vi "CreateLocationNode.vi"(7 "DOM Document":refnum<k20>, 8 "Error In":errorcluster, 11 "Pattern":string) -> (0 "Error Out":errorcluster, 3 "Location Node":refnum<k20>)   [LabVIEW 2012]
uses:
  libs/LV-Utilities/LV-Utilities.lvlib
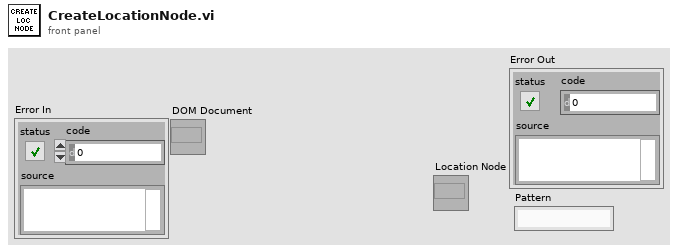
[diagram p1: front panel]
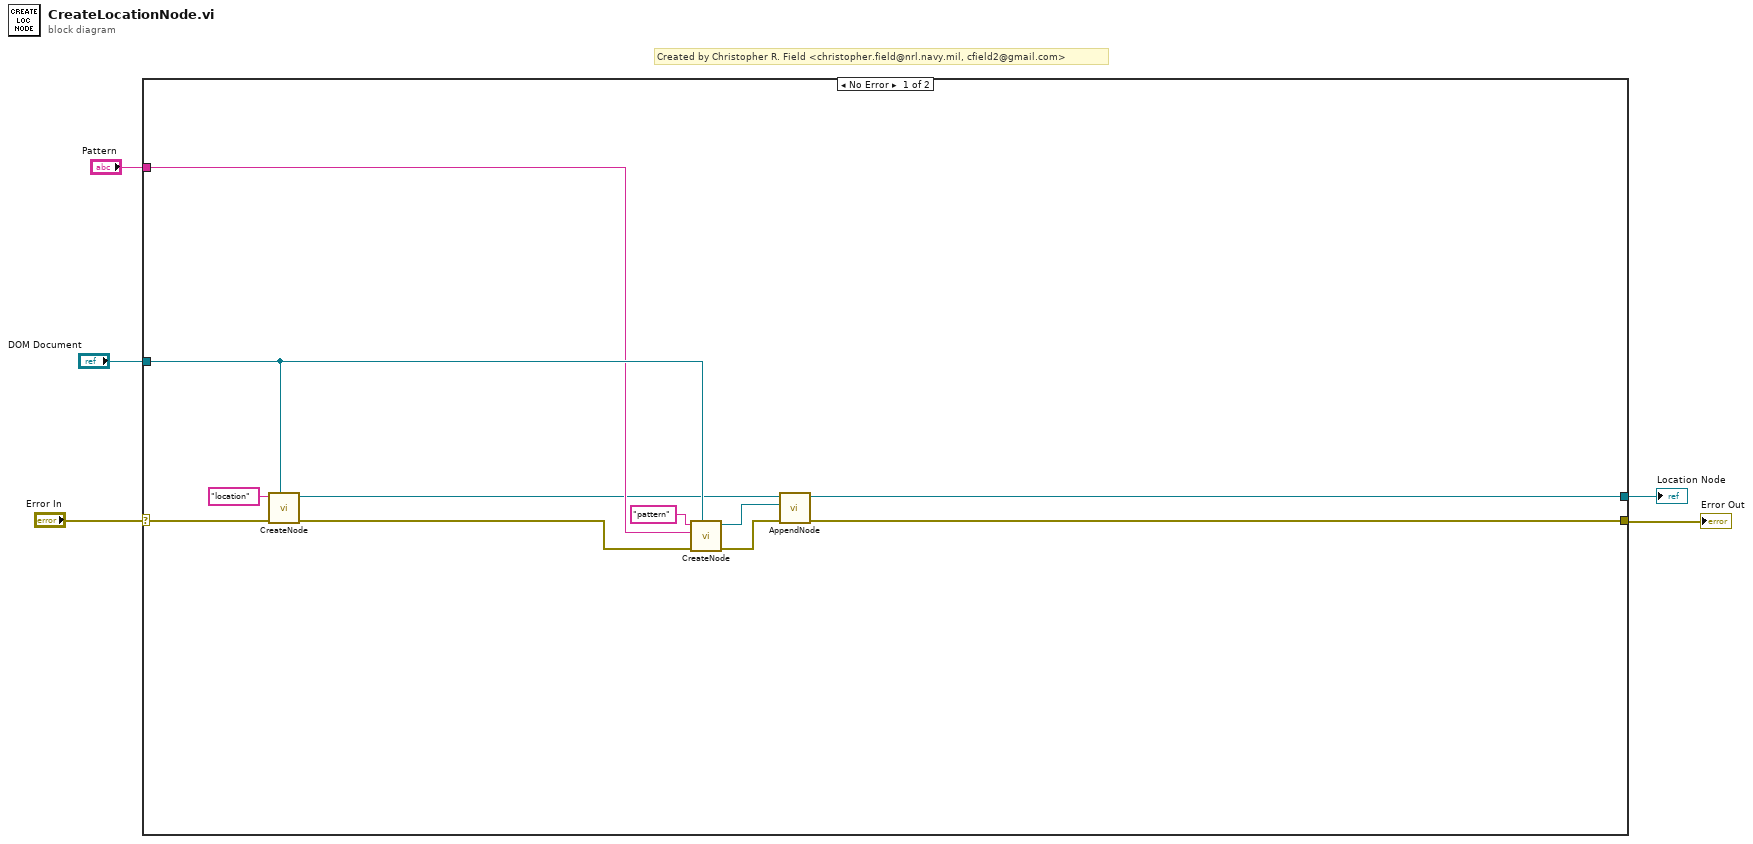
[diagram p0: block diagram]
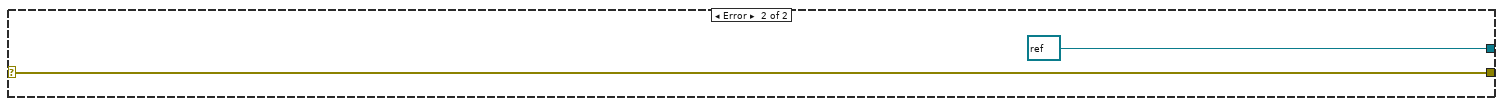
[diagram p2: hidden frame]
diagram:
  # "Created by Christopher R. Field <christopher.field@nrl.navy.mil, cfield2@gmail.com>"
  n1 = case shown="No Error" "Error In" {
    selector: "Error In" -> [w16 w18]
    tunnel: "DOM Document" -> [w14 _]
    tunnel: [w9 w18] -> w3
    tunnel: "Pattern" -> [w10 _]
    tunnel: [w8 refnum<k20> refnum ("Wirings Node 2")] -> w1
    frame No Error {
      n2 = call "CreateNode.vi"("DOM Document"=w14, "Error In"=w16, "Tag Name"="location") -> ("Error out"=w6:errorcluster, "Node"=w7:refnum<k20>)  [unwired: 7 in]
      n3 = call "CreateNode.vi"("DOM Document"=w14, "Error In"=w6, "Text"=w10, "Tag Name"="pattern") -> ("Error out"=w13:errorcluster, "Node"=w12:refnum<k20>)  [unwired: 6 in]
      n4 = call "AppendNode.vi"("Error In"=w13, "Child Node"=w12, "Parent Node In"=w7) -> ("Error Out"=w9:errorcluster, "Parent Node Out"=w8:refnum<k20>)  [unwired: 7 in]
    }
    frame Error {
    }
  }
  "Location Node" <- w1
  "Error Out" <- w3
